vi "BoxMullertest.vi"(8 "error in (no error)":errorcluster, 11 "RSA in":refnum<class "RSA.lvclass">) -> (0 "error out":errorcluster, 3 "RSA out":refnum<class "RSA.lvclass">)   [LabVIEW 2012, in "RSA.lvclass"]
uses:
  RSA.lvclass
  <vilib>/Analysis/NI_AALBase.lvlib
panel:
  out "standard deviation":dbl format="%0.2f"
  out "mean":dbl format="%0.2f"
  in  "x":dbl
  out "Histogram Graph":T1(graph)
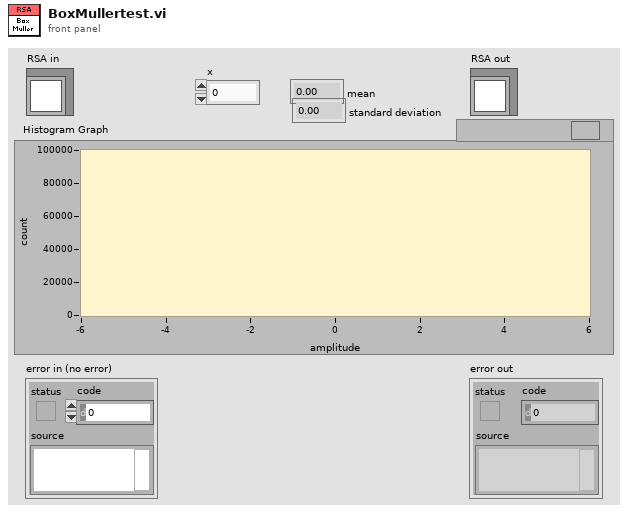
[diagram p1: front panel]
types:
  T1 = cluster{"X Values":dbl[], "Histogram: h(x)":i32[]}
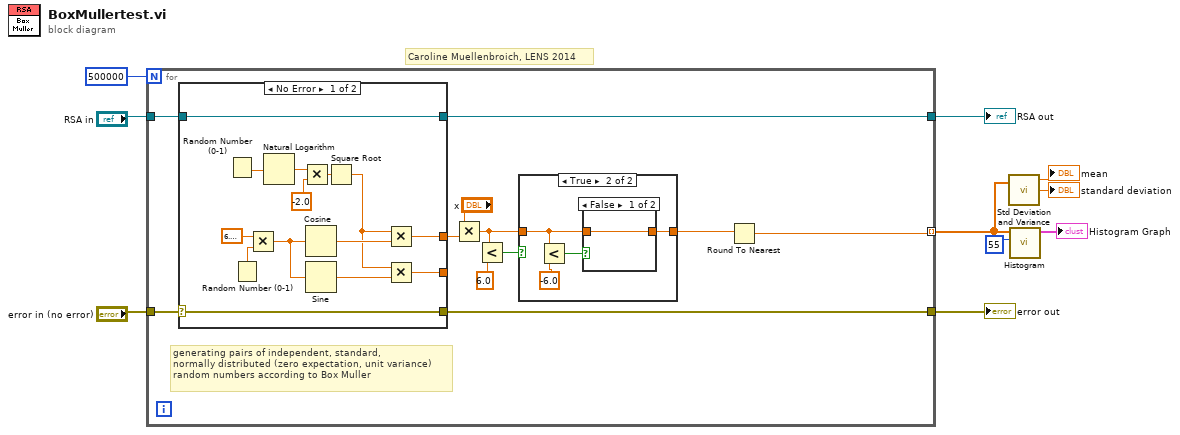
[diagram p0: block diagram]
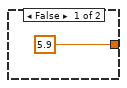
[diagram p2: hidden frame]
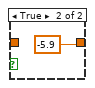
[diagram p3: hidden frame]
diagram:
  # "Caroline Muellenbroich, LENS 2014"
  n1 = for {
    N: 500000 -> [_]
    tunnel: [w11] -> w3 mode=indexing
    tunnel: [w21] -> w10
    tunnel: "error in (no error)" -> [w20]
    tunnel: "RSA in" -> [w19]
    tunnel: [w16] -> w4
    # "generating pairs of independent, standard,\nnormally distributed (zero expectation, unit variance)\nrandom numbers according to Box Muller"
    n2 = case shown="No Error" w20 {
      selector: w20 -> [w41 w44]
      tunnel: [w41 w44] -> w16
      tunnel: [w42 w43] -> w21
      tunnel: w19 -> [w42 w43]
      tunnel: [w30 _] -> w18
      tunnel: [w29 _] -> _
      frame No Error {
        n3 = Random Number (0-1)() -> (number: 0 to 1=w38:dbl)
        n4 = Random Number (0-1)() -> (number: 0 to 1=w36:dbl)
        n5 = Multiply(x=6.283185307179586, y=w36) -> (x*y=w33:dbl)
        n6 = Natural Logarithm(1:w38) -> (0:w39:dbl)
        n7 = Multiply(x=w39, y=-2.0 ("x")) -> (x*y=w37:dbl)
        n8 = Cosine(x=w33) -> (cos(x)=w34:dbl)
        n9 = Sine(x=w33) -> (sin(x)=w32:dbl)
        n10 = Square Root(x=w37) -> (sqrt(x)=w31:dbl)
        n11 = Multiply(x=w31, y=w34) -> (x*y=w30:dbl)
        n12 = Multiply(x=w31, y=w32) -> (x*y=w29:dbl)
      }
      frame Error {
      }
    }
    n13 = Multiply(x="x", y=w18) -> (x*y=w13:dbl)
    n14 = Less?(x=w13, y=6.0) -> (x < y?=w14:bool)
    n15 = case shown="True" w14 {
      tunnel: [5.9 w24] -> w12
      tunnel: w13 -> [_ w23]
      frame False {
      }
      frame True {
        n16 = Less?(x=w23, y=-6.0) -> (x < y?=w26:bool)
        n17 = case shown="False" w26 {
          tunnel: [w27 -5.9 ("y")] -> w24
          tunnel: w23 -> [w27 _]
          frame False {
          }
          frame True {
          }
        }
      }
    }
    n18 = Round To Nearest(number=w12) -> (nearest integer value=w11:dbl)
  }
  "RSA out" <- w10
  "error out" <- w4
  n19 = call <vilib>:"Std Deviation and Variance.vi"("X"=w3) -> ("mean"=→"mean":dbl, "standard deviation"=→"standard deviation":dbl)  [unwired: 1 in, 1 out]
  n20 = call <vilib>:"Histogram.vi"("intervals"=55, "X"=w3) -> ("Histogram Graph"=→"Histogram Graph":T1)  [unwired: 6 in, 3 out]
